vi "TEMPLATE Input.vi"(6 "Teller":refnum<data-value>, 8 "Error in":errorcluster, 10 "Input in":refnum<data-value>, 11 "TEMPLATE jettl Msg in":refnum<class "TEMPLATE jettl Msg.lvclass">) -> (0 "Error out":errorcluster, 2 "Input out":refnum<data-value>, 3 "TEMPLATE jettl Msg out":refnum<class "TEMPLATE jettl Msg.lvclass">)   [LabVIEW 2020, in "_Template.lvlib" / "Templates.lvlib" / "TEMPLATE jettl Msg.lvlib" / "TEMPLATE jettl Msg.lvclass"]
uses:
  TEMPLATE jettl Msg.lvclass
  jettl/jettl/Transport/Transport.lvclass
  jettl/jettl/Relation.ctl
  jettl/jettl/jettl.lvlib
  jettl/jettl/Teller.ctl
  Input.ctl
  TEMPLATE jettl Msg.lvlib
  jettl/jettl/Actor/Actor.lvclass
  jettl/jettl/Msg/Msg.lvclass
  jettl/jettl/Msgs.ctl
  jettl/jettl/Unified Layer.ctl
  jettl/jettl/Actor Attributes.ctl
panel:
  # "This front panel should not be manipulated."
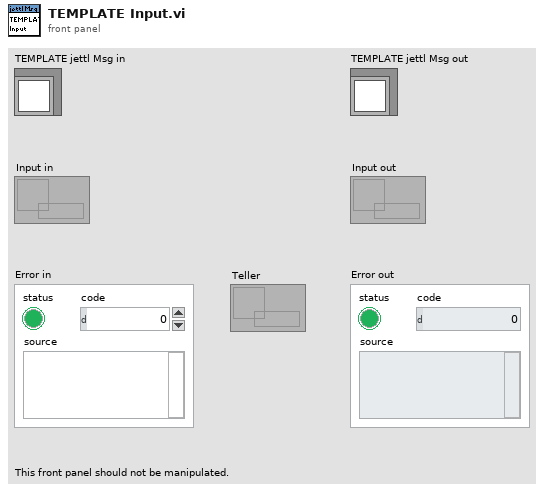
[diagram p1: front panel]
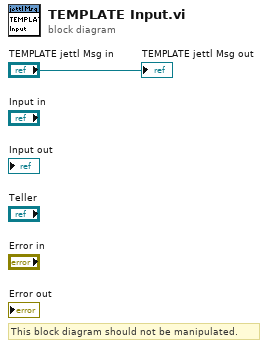
[diagram p0: block diagram]
diagram:
  # "This block diagram should not be manipulated."
  "TEMPLATE jettl Msg out" <- "TEMPLATE jettl Msg in"
